vi "Voltage_global.vi"() -> ()   [LabVIEW 2015]
panel:
  out "MyInterruptVoltage":dbl
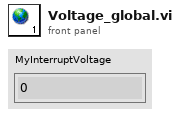
[diagram p1: front panel]
diagram:
